vi "match_secondary_file.vi"(8 "secondary":string, 11 "string array in":string[](array[string])) -> (3 "string array out":string[](array[string]))   [LabVIEW 2017]
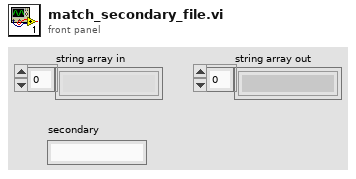
[diagram p1: front panel]
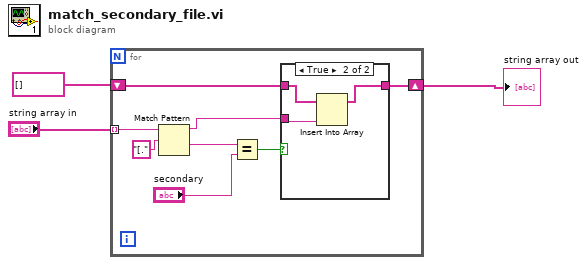
[diagram p0: block diagram]
diagram:
  n1 = for {
    tunnel: "string array in" -> [w6] mode=indexing
    shift-right: [w8] -> w3
    shift-left: string[] [] ("filenames") -> [w9]
    n2 = Match Pattern(string=w6, regular expression="[.") -> (before substring=w4:string, after substring=w7:string)  [unwired: 1 in, 2 out]
    n3 = Equal?(x=w7, y="secondary") -> (x = y?=w10:bool)
    n4 = case shown="True" w10 {
      tunnel: w9 -> [w12 w14]
      tunnel: [w12 w13] -> w8
      tunnel: w4 -> [_ w15]
      frame False {
      }
      frame True {
        n5 = Insert Into Array(array=w14, new element=w15) -> (w13:string[])  [unwired: 1 in]
      }
    }
  }
  "string array out" <- w3
